vi "DigInputs Write.vi"(4 "error in (no error)":errorcluster, 5 "Value":string[](array[string]), 6 "Container State":T3, 7 "Display State In":T1) -> (0 "error out":errorcluster, 3 "Display State Out":T1)   [LabVIEW 2020, in "Input Criterion.xctl"]
uses:
  Input Criterion.xctl
  <vilib>/_xctls/Container State.ctl
  State.vi
  Events.ctl
  Event Type.ctl
  Operator.vi
  Digital Input VIs/Tosca-Input Criterion.ctl
  epl-vi-lib/Utility VIs/Type Defs/Logic State.ctl
  <vilib>/_xctls/XControlSupport.lvlib
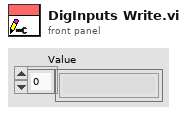
[diagram p1: front panel]
types:
  T1 = typedef "Input Criterion.xctl/State.vi" = cluster{"DI":string[], "Flags":string[], "show op":bool, "flag start":i16, "Events":T2}
  T2 = typedef "Input Criterion.xctl/Events.ctl" = cluster{"Generic":refnum<user-event>, "Operator":refnum<user-event>, "Criterion":refnum<user-event>}
  T3 = typedef "XControlSupport.lvlib/Container State.ctl" = cluster{"Indicator?":bool, "Run Mode?":bool, " Refnum":refnum<vi>}
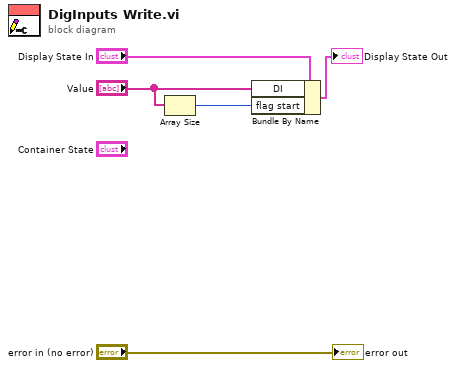
[diagram p0: block diagram]
diagram:
  n1 = Array Size(array="Value") -> (size(s)=w1:i32)
  n2 = Bundle By Name(cluster="Display State In", "DI"="Value", "flag start"=w1) -> (→"Display State Out":T1)
  "error out" <- "error in (no error)"
